vi "GetMeasurements.vi"(8 "error in (no error)":errorcluster, 11 "ByteGSAPIBase in":refnum<class "ByteGSAPIBase.lvclass">) -> (0 "error out":errorcluster, 2 "measurements":T1(array[cluster]), 3 "ByteGSAPIBase out":refnum<class "ByteGSAPIBase.lvclass">)   [LabVIEW 2019, in "ByteGSWebAPI.lvlib" / "ByteGSAPIBase.lvclass"]
doc: "Obtain all measurements"
uses:
  ByteGSAPIBase.lvclass
  TypeDef/EditMeasurementReqData.ctl
  ByteGSAPIBase.lvclass/ByteGSAPIBase.ctl
  <vilib>/Bytelabs/ByteREST/ByteRESTClass/ByteRESTBase/RESTBase.lvclass
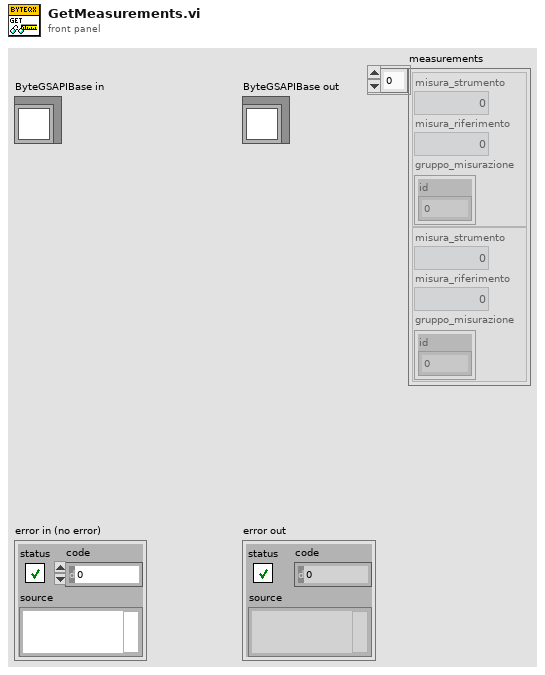
[diagram p1: front panel]
types:
  T1 = cluster{"misura_strumento":sgl, "misura_riferimento":sgl, "gruppo_misurazione":cluster{"id":i32}}[]
  T2 = typedef "ByteGSWebAPI.lvlib/ByteGSAPIBase.lvclass/EditMeasurementReqData.ctl" = cluster{"Id_Group":i32, "misura_strumento":sgl, "misura_riferimento":sgl}
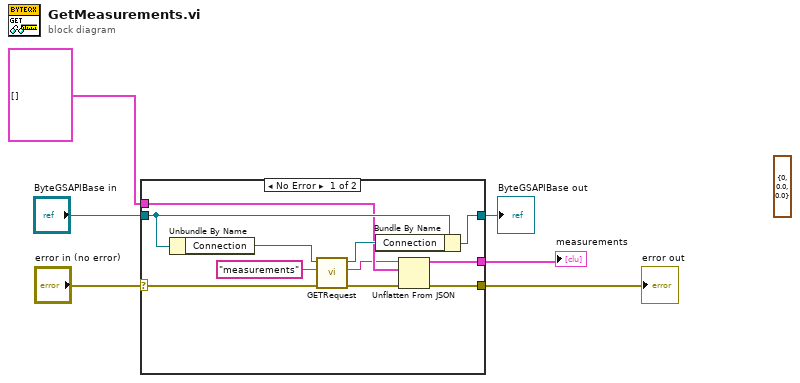
[diagram p0: block diagram]
diagram:
  (unwired) T2 {"Id_Group"=0, "misura_strumento"=0.0, "misura_riferimento"=0.0} ("Valori")
  n1 = case shown="No Error" "error in (no error)" {
    selector: "error in (no error)" -> [w11 w20]
    tunnel: [w10 w20] -> w4
    tunnel: T1 [] ("Valori") -> [w9 w19]
    tunnel: [w8 w19] -> w2
    tunnel: [w14 w18] -> w5
    tunnel: "ByteGSAPIBase in" -> [w17 w18]
    frame No Error {
      n2 = Unbundle By Name(w17) -> ("Connection"=w16:refnum<class "RESTBase.lvclass">)
      n3 = call-dynamic "GETRequest.vi"("error in (no error)"=w11, "Request"="measurements", "ByteRESTBase in"=w16) -> ("error out"=w15:errorcluster, "Body"=w7:string, "ByteRESTBase out"=w13:refnum<class "RESTBase.lvclass">)  [unwired: 5 in, 1 out]
      n4 = Bundle By Name(cluster=w17, "Connection"=w13) -> (w14:refnum<class "ByteGSAPIBase.lvclass">)
      n5 = Unflatten From JSON(JSON string=w7, type and defaults=w9, error in (no error)=w15) -> (value=w8:T1, error out=w10:errorcluster)  [unwired: 4 in]
    }
    frame Error {
    }
  }
  "error out" <- w4
  "ByteGSAPIBase out" <- w5
  "measurements" <- w2
